vi "1L23_conv_Kelvin_degre.vi"(1 "Deg K":dbl format="%.2f") -> (0 "Deg C":dbl format="%.2f")   [LabVIEW 2010, in "lv_01.lvlib"]
doc: "Conversion de degré Kelvin en Celsius."
uses:
  lv_01.lvlib
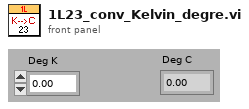
[diagram p1: front panel]
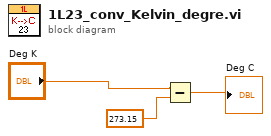
[diagram p0: block diagram]
diagram:
  n1 = Subtract(x="Deg K", y=273.15) -> (x-y=→"Deg C":dbl)
